vi "Test Log.vi"() -> ()   [LabVIEW 2014, in "System Log.lvclass"]
uses:
  System Log.lvclass
  <userlib>/_Session Fwk/Session - Root.lvclass
panel:
  in  "showFP":bool
  out "error out 2":errorcluster
  out "error out":errorcluster
  in  "logevent":bool
  in  "error in":errorcluster
  in  "Msg":string
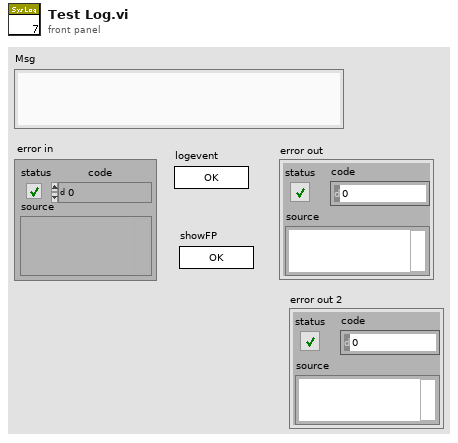
[diagram p1: front panel]
types:
  T1 = typedef "Session - Root.lvclass/Session Handle.ctl" = refnum<data-value>
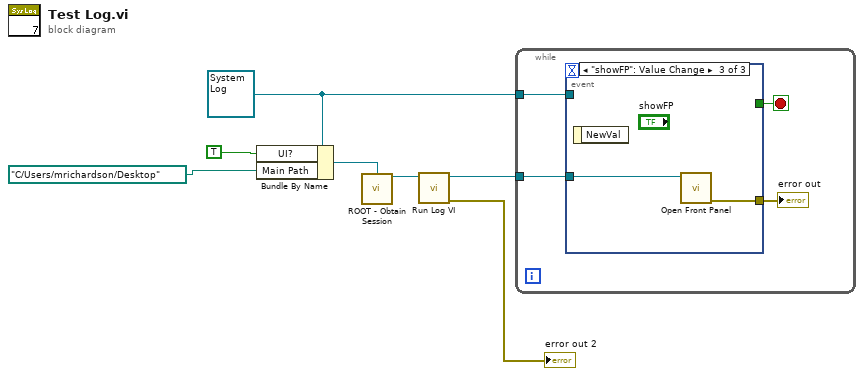
[diagram p0: block diagram]
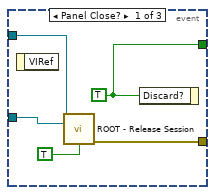
[diagram p2: hidden frame]
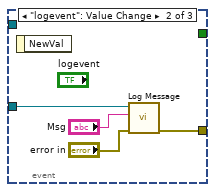
[diagram p3: hidden frame]
diagram:
  w4 = refnum<class "System Log.lvclass"> refnum ("Sys Log")
  n1 = Bundle By Name(cluster=w4, "UI?"=TRUE, "Main Path"=path "C:/Users/mrichardson/Desktop") -> (w5:refnum<class "System Log.lvclass">)
  n2 = call <userlib>:"ROOT - Obtain Session.vi"("OBJ - Session"=w5) -> ("Session Handle"=w3:T1)  [unwired: 12 in, 2 out]
  n3 = call "Run Log VI.vi"("Session Handle In"=w3) -> ("error out"=→"error out 2":errorcluster, "Session Handle Out"=w2:T1)  [unwired: 9 in]
  n4 = while {
    tunnel: w2 -> [w10]
    tunnel: w4 -> [w9]
    stop <- w11 stop-if-true
    n5 = event shown="[2] \"showFP\": Value Change" {
      selector: _ -> [_ _ _]
      dyn-events: _ -> [_ _ _]
      timeout: _ -> [_ _ _]
      tunnel: [w16 _ _] -> w11
      tunnel: w10 -> [w15 w17 w22]
      tunnel: w9 -> [w14 _ _]
      tunnel: [w13 w18 w21] -> w8
      event Panel Close? {
        w16 = TRUE ("Discard?")
        n6 = event-data() -> ()  [unwired: 1 in, 1 out]
        n7 = call <userlib>:"ROOT - Release Session.vi"("OBJ - Session in"=w14, "Session Handle in"=w15, "force destroy? (F)"=TRUE) -> ("error out"=w13:errorcluster)  [unwired: 11 in, 1 out]
        n8 = event-data("Discard?"=w16) -> ()  [unwired: 1 in, 1 out]
      }
      event "logevent": Value Change {
        n9 = event-data() -> ()  [unwired: 1 in, 1 out]
        n10 = call "Log Message.vi"("error in"="error in", "MSG In"="Msg", "session in"=w17) -> ("error out"=w18:errorcluster)  [unwired: 7 in, 1 out]
      }
      event "showFP": Value Change {
        n11 = event-data() -> ()  [unwired: 1 in, 1 out]
        n12 = call "Open Front Panel.vi"("Session In"=w22) -> ("error out"=w21:errorcluster)  [unwired: 9 in, 1 out]
      }
    }
    "error out" <- w8
  }
